vi "Protocolo_DI.vi"(3 "Trama2":i8, 5 "Trama1":i8) -> (0 "Digital2":bool, 1 "Digital1":bool, 2 "Analogico":u32)   [LabVIEW 2017]
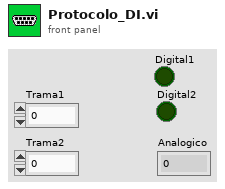
[diagram p1: front panel]
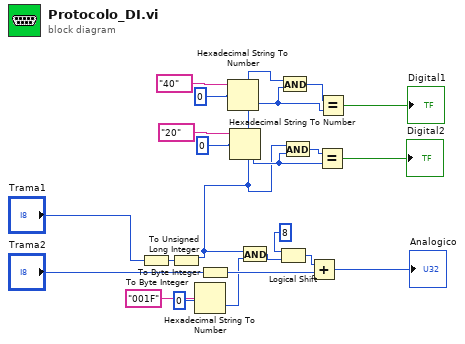
[diagram p0: block diagram]
diagram:
  n1 = To Byte Integer(number="Trama1") -> (8bit integer=w22:i8)
  n2 = To Unsigned Long Integer(number=w22) -> (unsigned 32bit integer=w7:u32)
  n3 = Hexadecimal String To Number(string="001F", offset=0) -> (number=w8:u32)  [unwired: 1 in, 1 out]
  n4 = To Byte Integer(number="Trama2") -> (8bit integer=w21:i8)
  n5 = Hexadecimal String To Number(string="40", offset=0) -> (number=w13:u32)  [unwired: 1 in, 1 out]
  n6 = Hexadecimal String To Number(string="20", offset=0) -> (number=w14:u32)  [unwired: 1 in, 1 out]
  n7 = And(x=w7, y=w8) -> (x .and. y?=w6:u32)
  n8 = Logical Shift(y=8, x=w6) -> (x << y=w11:u32)
  n9 = And(x=w7, y=w13) -> (x .and. y?=w15:u32)
  n10 = And(x=w7, y=w14) -> (x .and. y?=w16:u32)
  n11 = Add(x=w11, y=w21) -> (x+y=→"Analogico":u32)
  n12 = Equal?(x=w16, y=w14) -> (x = y?=→"Digital2":bool)
  n13 = Equal?(x=w15, y=w13) -> (x = y?=→"Digital1":bool)
